vi "VCS Get Analog Input.vi"(8 "error in (no error)":errorcluster, 10 "number":u16=1, 11 "axis in":cluster{"keyHandle":u32, "nodeId":u16}={"keyHandle"=0, "nodeId"=1}) -> (0 "error out":errorcluster, 2 "analogInput":u16, 3 "axis out":cluster{"keyHandle":u32, "nodeId":u16}={"keyHandle"=0, "nodeId"=1})   [LabVIEW 2018]
doc: "<B>VCS Get Analog Input</B> returns the analog value from selected input."
uses:
  Resources/EposCmd.dll
  Resources/EposCmd64.dll
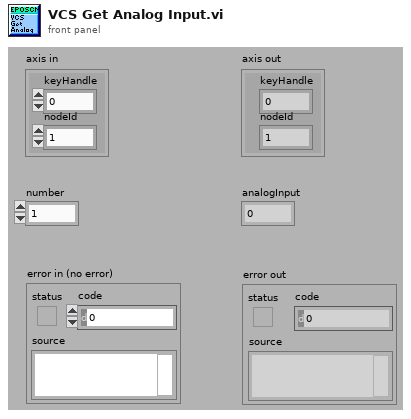
[diagram p1: front panel]
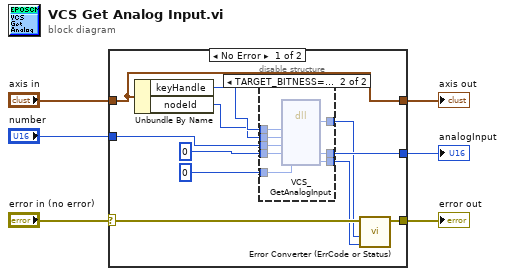
[diagram p0: block diagram]
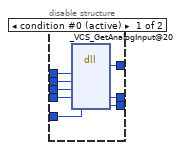
[diagram p2: hidden frame]
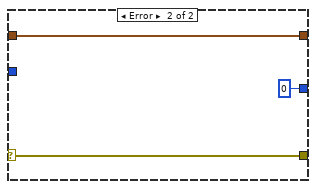
[diagram p3: hidden frame]
diagram:
  n1 = case shown="No Error" "error in (no error)" {
    selector: "error in (no error)" -> [w15 w36]
    tunnel: [w14 w36] -> w5
    tunnel: "number" -> [w17 _]
    tunnel: [w16 u16 0 ("pAnalog")] -> w3
    tunnel: "axis in" -> [w8 w35]
    tunnel: [w8 w35] -> w1
    frame No Error {
      n2 = Unbundle By Name(w8) -> ("keyHandle"=w12:u32, "nodeId"=w11:u16)
      n3 = disable-structure shown="TARGET_BITNESS==64" {
        disable-tunnel: w17 -> [w25 w33]
        disable-tunnel: [w24 w32] -> w16
        disable-tunnel: [w23 w31] -> w13
        disable-tunnel: w12 -> [w22 w30]
        disable-tunnel: w11 -> [w21 w29]
        disable-tunnel: u16 0 ("pAnalog") -> [w20 w28]
        disable-tunnel: u32 0 ("pErrorCode") -> [w19 w27]
        disable-tunnel: [w18 w26] -> w7
        frame condition #0 (active) {
          n4 = dll-call lib="C:/Projeto em LabVIEW/EPOS-LabVIEW-Instrument-Driver-En/LabVIEW/maxon EPOS/Resources/EposCmd.*" fn="_VCS_GetAnalogInput@20"("KeyHandle"=w22, "NodeId"=w21, "Number"=w25, "pAnalog"=w20, "pErrorCode"=w19) -> (w18:i32, "pAnalog"=w24:u16, "pErrorCode"=w23:u32)  [unwired: 6 in, 2 out]
        }
        frame condition #1 {
          n5 = dll-call lib="C:/setup/Resources/EposCmd64.*" fn="VCS_GetAnalogInput" ("EposCmd.dll:_VCS_GetAnalogInput@20")("KeyHandle"=w30, "NodeId"=w29, "Number"=w33, "pAnalog"=w28, "pErrorCode"=w27) -> ("Rückgabetyp"=w26:i32, "pAnalog"=w32:u16, "pErrorCode"=w31:u32)  [unwired: 6 in, 2 out]
        }
      }
      n6 = call "Error Converter (ErrCode or Status).vi"("error code"=w13, "return type"=w7, "error in (no error)"=w15) -> ("error out"=w14:errorcluster)  [unwired: 7 in]
    }
    frame Error {
    }
  }
  "analogInput" <- w3
  "error out" <- w5
  "axis out" <- w1
